vi "create Paycheck.vi"(5 "Account":string, 7 "Date":timestamp, 8 "error in (no error)":errorcluster, 9 "Amount":dbl, 10 "Job":string, 11 "Paycheck in":refnum<class "Paycheck.lvclass">) -> (0 "error out":errorcluster, 3 "Paycheck out":refnum<class "Paycheck.lvclass">)   [LabVIEW 2020, in "Paycheck.lvclass"]
uses:
  Paycheck.lvclass
  Paycheck.lvclass/Paycheck.ctl
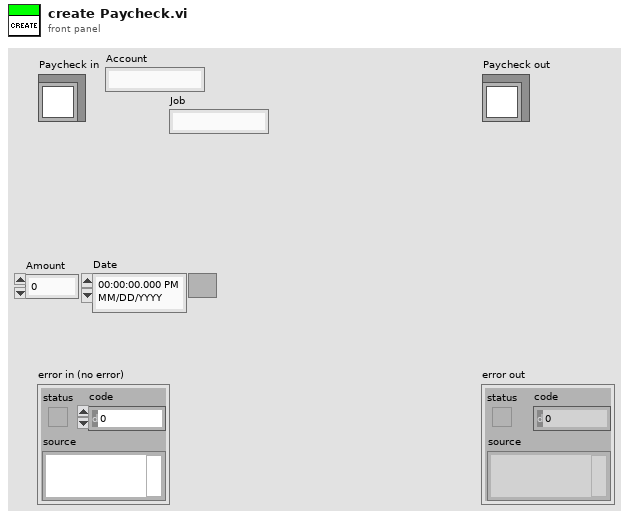
[diagram p1: front panel]
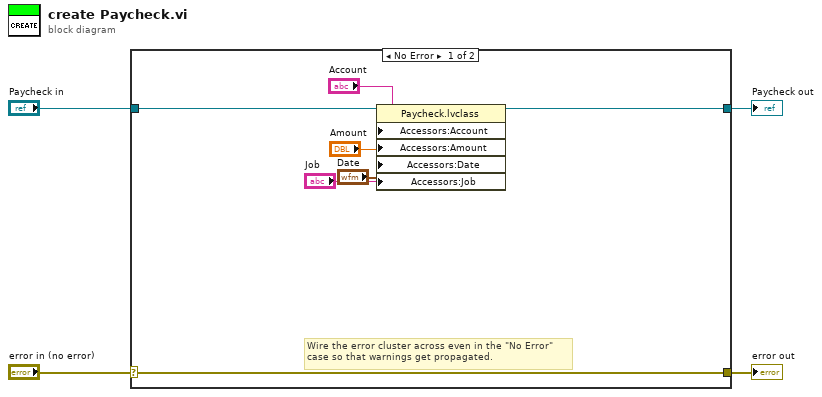
[diagram p0: block diagram]
diagram:
  n1 = case shown="No Error" "error in (no error)" {
    selector: "error in (no error)" -> [w10 w13]
    tunnel: [w10 w13] -> w3
    tunnel: [w9 w12] -> w1
    tunnel: "Paycheck in" -> [w11 w12]
    frame No Error {
      # "Wire the error cluster across even in the \"No Error\"\ncase so that warnings get propagated."
      n2 = property class="Paycheck.lvclass"(reference=w11, "Accessors:Account"="Account", "Accessors:Amount"="Amount", "Accessors:Date"="Date", "Accessors:Job"="Job") -> (reference out=w9:refnum<class "Paycheck.lvclass">)  [unwired: 1 in, 1 out]
    }
    frame Error {
    }
  }
  "error out" <- w3
  "Paycheck out" <- w1
